vi "PmacButtSendStr.vi"(1 "Button State Bool":bool, 2 "Command String":string, 3 "Device Number i32 (0)":i32 min=0) -> (0 "Response Available Bool (F)":bool)   [LabVIEW 2020]
doc: "Send Command String to PMAC when Button State is TRUE. Response Available is TRUE when PMAC has processed the command."
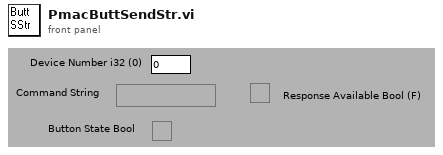
[diagram p1: front panel]
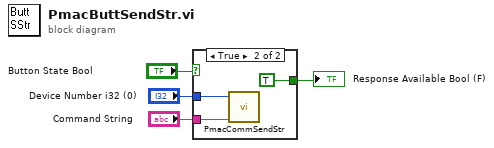
[diagram p0: block diagram]
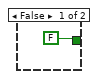
[diagram p2: hidden frame]
diagram:
  n1 = case shown="True" "Button State Bool" {
    tunnel: "Command String" -> [_ w8]
    tunnel: "Device Number i32 (0)" -> [_ w7]
    tunnel: [FALSE TRUE ("Button State Bool (F)")] -> w1
    frame False {
    }
    frame True {
      n2 = call "PmacCommSendStr.vi"("Command String"=w8, "Device Number i32 (0)"=w7) -> ()  [unwired: 1 out]
    }
  }
  "Response Available Bool (F)" <- w1
